vi "Parse Syntax Text.vi"(8 "error in (no error)":errorcluster, 10 "Segment":T1, 11 "ProtoParser in":refnum<class "ProtoParser.lvclass">) -> (0 "error out":errorcluster, 2 "Syntax":T3, 3 "ProtoParser out":refnum<class "ProtoParser.lvclass">)   [LabVIEW 2020, in "LV-Protoc.lvlib" / "ProtoParser.lvclass"]
uses:
  ProtoParser.lvclass
  Syntax.ctl
  LV-Protoc.lvlib
  Segment Type.ctl
  Raw Segment.ctl
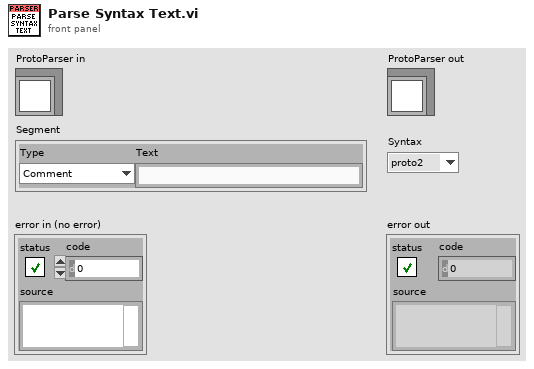
[diagram p1: front panel]
types:
  T1 = typedef "LV-Protoc.lvlib/Raw Segment.ctl" = cluster{"Type":T2, "Text":string}
  T2 = typedef "LV-Protoc.lvlib/Segment Type.ctl" = enum16{"Comment", "Message Open", "Enum Open", "Message Close", "Enum Close", "Field", "Syntax", "Import", "Enum Value", "Package", "Reserved"}
  T3 = typedef "LV-Protoc.lvlib/Syntax.ctl" = enum16{"proto2", "proto3"}
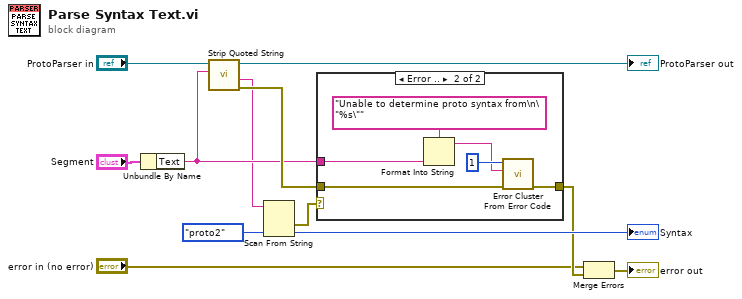
[diagram p0: block diagram]
diagram:
  n1 = Unbundle By Name("Segment") -> ("Text"=w3:string)
  n2 = call "Strip Quoted String.vi"("Text"=w3, "ProtoParser in"="ProtoParser in") -> ("error out"=w12:errorcluster, "String Contents"=w1:string, "ProtoParser out"=→"ProtoParser out":refnum<class "ProtoParser.lvclass">)  [unwired: 6 in, 1 out]
  n3 = Scan From String(input string=w1, default 1=Syntax."proto2" ("Syntax")) -> (error out=w8:errorcluster, output 1=→"Syntax":T3)  [unwired: 3 in, 2 out]
  n4 = case shown="Error .." w8 {
    tunnel: w12 -> [w13 w19]
    tunnel: [w13 w18] -> w7
    tunnel: w3 -> [_ w16]
    frame No Error {
    }
    frame Error {
      n5 = Format Into String(format string="Unable to determine proto syntax from\n\"%s\"", w16) -> (resulting string=w15:string)  [unwired: 2 in, 1 out]
      n6 = call <vilib>:"Error Cluster From Error Code.vi"("error in (no error)"=w19, "error message (\"\")"=w15, "error code (0)"=1) -> ("error out"=w18:errorcluster)  [unwired: 6 in]
    }
  }
  n7 = Merge Errors("error in (no error)", w7) -> (→"error out":errorcluster)
